vi "Write Cell Frequency Data.vi"(8 "error in":errorcluster, 10 "freqData":waveform(dbl), 11 "PAS Data in":refnum<class "PAS Data.lvclass">=refnum) -> (0 "error out":errorcluster, 3 "PAS Data out":refnum<class "PAS Data.lvclass">)   [LabVIEW 2014, in "PAS Data.lvclass"]
uses:
  PAS Data.lvclass
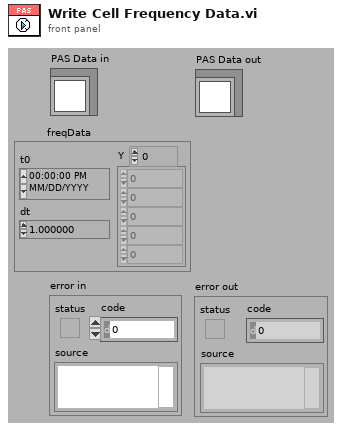
[diagram p1: front panel]
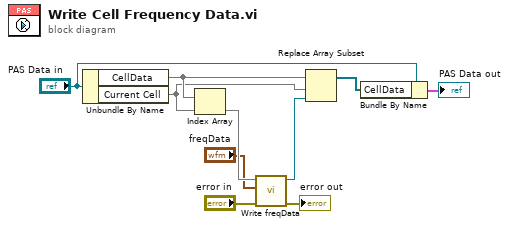
[diagram p0: block diagram]
diagram:
  n1 = Unbundle By Name("PAS Data in") -> ("CellData"=w7, "Current Cell"=w5)
  n2 = Index Array(array=w7, index=w5) -> (element=w10)
  n3 = call "Write freqData.vi"("error in (no error)"="error in", "freqData"="freqData", "PAS Cell Data in"=w10) -> ("error out"=→"error out":errorcluster, "PAS Cell Data out"=w6:refnum<class "PAS Cell Data.lvclass">)  [unwired: 7 in]
  n4 = Replace Array Subset(array=w7, new element=w6, index=w5) -> (w3:refnum<class "PAS Cell Data.lvclass">[])
  n5 = Bundle By Name(cluster="PAS Data in", "CellData"=w3) -> (→"PAS Data out":cluster{})
